vi "visn_Calculate CRC-5 (Bits Array)Fer.vi"(11 "Bits Array":u8[](array[numeric])=[1, 1, 0, 0, 1, 1, 1, 0, 1, 0] format="%0x") -> (3 "CRC-5":u8[](array[numeric])=[1, 1, 0, 0, 1] format="%0x")   [LabVIEW 2015]
panel:
  out "loop":i32
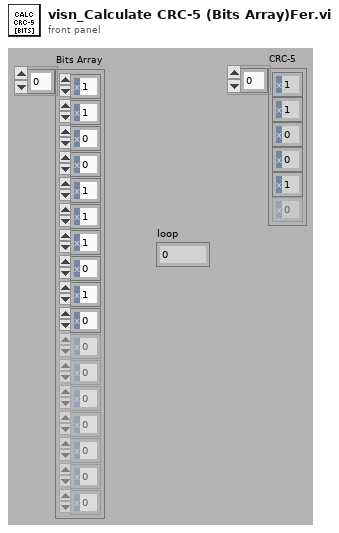
[diagram p1: front panel]
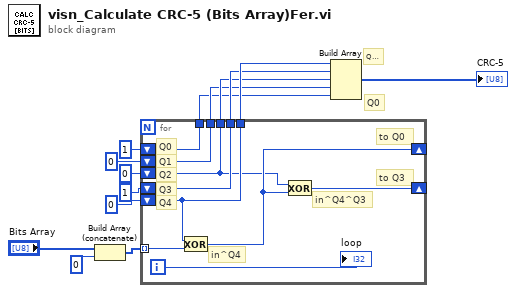
[diagram p0: block diagram]
diagram:
  # "QQ4"
  # "Q0"
  n1 = Build Array (concatenate)("Bits Array", u8 0) -> (w3:u8[])
  n2 = for {
    shift-right: [w22] -> _
    shift-left: u8 0 -> [w17]
    shift-left: u8 0 -> [w18]
    tunnel: w3 -> [w23] mode=indexing
    shift-right: [w21] -> _
    shift-left: u8 0 -> [w20]
    shift-left: u8 1 -> [w16]
    shift-left: u8 1 -> [w19]
    tunnel: [w20] -> w9
    tunnel: [w19] -> w8
    tunnel: [w18] -> w7
    tunnel: [w17] -> w6
    tunnel: [w16] -> w5
    i -> [w15]
    # "Q1"
    # "Q2"
    # "Q3"
    # "Q4"
    # "to Q3"
    # "to Q0"
    # "in^Q4^Q3"
    # "in^Q4"
    # "Q0"
    n3 = Exclusive Or(1:w23, 2:w20) -> (0:w22:u8)
    n4 = Exclusive Or(1:w22, 2:w18) -> (0:w21:u8)
    "loop" <- w15
  }
  n5 = Build Array(w9, w8, w7, w6, w5) -> (→"CRC-5":u8[])
